vi "myRIO_PWM_Decoder.vi"() -> ()   [LabVIEW 2013]
doc: "https://decibel.ni.com/content/docs/DOC-30483"
uses:
  <vilib>/Platform/TimedLoop/XDataNode/timing_clust.ctl
  <vilib>/Platform/TimedLoop/XDataNode/nitl_modes.ctl
  <vilib>/Platform/TimedLoop/XDataNode/wakeup.ctl
  <vilib>/rvi/Emulation/niFpgaSctlEmulationGetInTimedLoop.vi
  <vilib>/rvi/Emulation/niFpgaEmulationReportErrorSimple.vi
  <vilib>/rvi/Emulation/niFpgaGetClockAttributes.vi
  <vilib>/rvi/Emulation/niFpgaCriticalErrorInLSC.vi
  <vilib>/rvi/eio/common/nirviEmuTemplateMethod_errors.vi
  <vilib>/Platform/TimedLoop/XDataNode/XDataNode.xnode
  <vilib>/eio/EIONode/EIONode.xnode
  <vilib>/Platform/TimedLoop/XDataNode/XDNodeRunTimeDep.lvlib
panel:
  out "Switch High Center":u32
  out "Rudder High Center":u32
  out "Sail High Center":u32
  out "Switch Low Center":u32
  out "Rudder Low Center":u32
  out "Sail Low Center":u32
  # "Connector A"
  # "Decoders"
  # "this VI measures the HIGH and LOW times of the given Digital Inputs on Connector A and B in order to measure the PWM duty cycles on the RT-side"
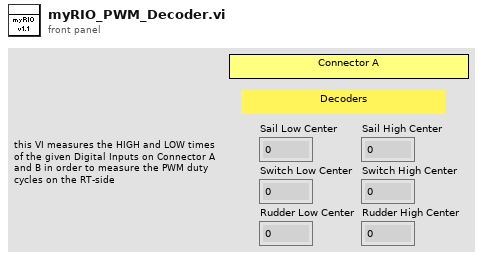
[diagram p1: front panel]
types:
  T1 = typedef "XDNodeRunTimeDep.lvlib/timing_clust.ctl" = cluster{"Expected End [f-1]":u64, "Actual End [f-1]":u64, "Finished Late? [f-1]":bool, "Expected End [i-1]":u64, "Actual End [i-1]":u64, "Finished Late? [i-1]":bool, "Expected Start [i]":u64, "Actual Start [i]":u64, "Expected Start [f]":u64, "Actual Start [f]":u64, "Source Name":string, "Structure Name":string, "Period":i64, "Deadline":i64, "Offset":i64, "Start":i64, "Priority":i32, "Timeout":i32, "Mode":T2, "Wakeup Reason":T3, "Error":errorcluster, "Source Type":string, "Secondary Source Type":string, "Global End Time":u64, "Global Start Time":u64, "Frame Duration":u64, "Iteration Duration":u64, "Assigned CPU":i32, "I/O Scan Engine Mode":u32}
  T2 = typedef "XDNodeRunTimeDep.lvlib/nitl_modes.ctl" = enum32{"No Change", "Process missed periods, maintain original phase", "Discard missed periods, maintain original phase", "Process missed periods, ignore original phase", "Discard missed periods, ignore original phase"}
  T3 = typedef "XDNodeRunTimeDep.lvlib/wakeup.ctl" = enum32{"Normal", "Aborted", "Asynchronous wakeup", "Timing source error", "Timed loop error", "Timeout"}
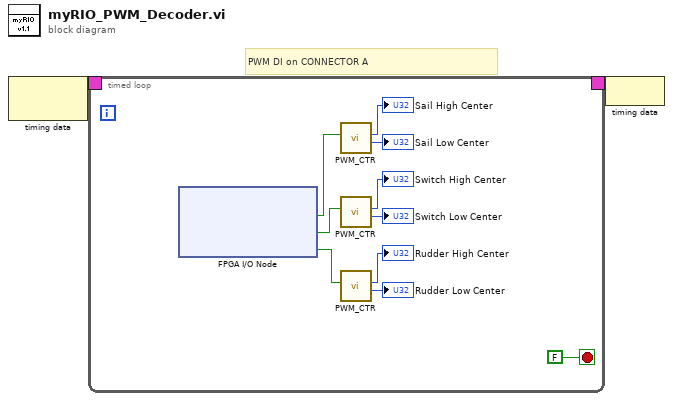
[diagram p0: block diagram]
diagram:
  # "PWM DI on CONNECTOR A"
  n1 = node-c288() -> (w2:T1)  [unwired: 1 in]
  n2 = timed-loop {
    timing: w2 -> [_]
    timing-out: [_] -> w1
    stop <- FALSE stop-if-true
    n3 = xnode "FPGA I/O Node"() -> ("ConnectorA/DIO0"=w12:bool, "ConnectorA/DIO1"=w11:bool, "ConnectorA/DIO2"=w10:bool)  [unwired: 3 in, 3 out]
    n4 = call "PWM_CTR.vi"("SIG_IN"=w12) -> ("LOW CTR"=→"Sail Low Center":u32, "HIGH CTR"=→"Sail High Center":u32)  [unwired: 9 in]
    n5 = call "PWM_CTR.vi"("SIG_IN"=w11) -> ("LOW CTR"=→"Switch Low Center":u32, "HIGH CTR"=→"Switch High Center":u32)  [unwired: 9 in]
    n6 = call "PWM_CTR.vi"("SIG_IN"=w10) -> ("LOW CTR"=→"Rudder Low Center":u32, "HIGH CTR"=→"Rudder High Center":u32)  [unwired: 9 in]
  }
  n7 = node-c288(w1) -> ()
